vi "CVT Action Engine.vi"() -> ()   [LabVIEW 2021]
uses:
  CVT Command.ctl
  CVT Data Highway.ctl
  <vilib>/NI/Current Value Table/Current Value Table.lvlib
  <vilib>/NI/Current Value Table/Type Defs/Data Types.ctl
  <vilib>/NI/Current Value Table/Type Defs/Single Tag.ctl
  <vilib>/NI/Current Value Table/Type Defs/Tag Grouping set.ctl
  <vilib>/NI/Current Value Table/Type Defs/File Format.ctl
  <vilib>/NI/Current Value Table/DataTypes/Boolean_Write.vi
panel:
  in  "CVT Command":T1
  out "error out":errorcluster
  in  "error in (no error)":errorcluster
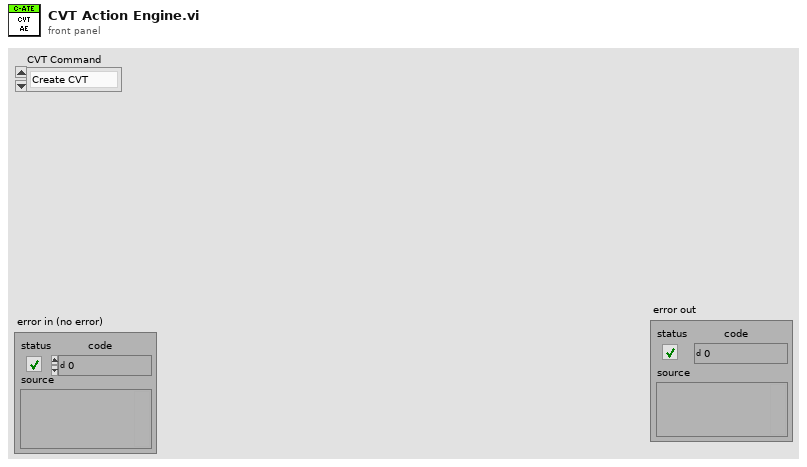
[diagram p1: front panel]
types:
  T1 = typedef "CVT Command.ctl" = enum16{"Create CVT", "Write Data ", "Read Data"}
  T2 = typedef "Current Value Table.lvlib/File Format.ctl" = cluster{"Tags":T3[], "Group Listings":T5[]}
  T3 = typedef "Current Value Table.lvlib/Single Tag.ctl" = cluster{"Data Type":T4, "Name":string, "Value":string, "Description":string}
  T4 = typedef "Current Value Table.lvlib/Data Types.ctl" = enum16{"Double", "Single", "I64", "I32", "I16", "I8", "U64", "U32", "U16", "U8", "String", "Boolean", "Array of U8", "Array of U16", "Array of U32", "Array of U64", "Array of I64", "Array of I32", "Array of I16", "Array of I8", "Array of Double", "Array of Single", "Array of Boolean", "Array of String"}
  T5 = typedef "Current Value Table.lvlib/Tag Grouping set.ctl" = cluster{"Group":string, "Tag Names":string[]}
  T6 = typedef "CVT Data Highway.ctl" = cluster{}
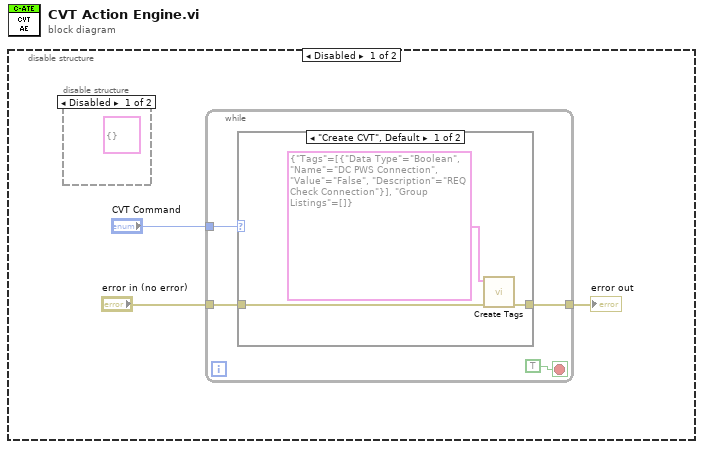
[diagram p0: block diagram]
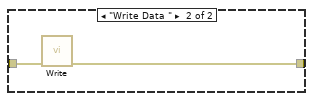
[diagram p3: hidden frame]
diagram:
  n1 = disable-structure shown="Disabled" {
    frame Disabled {
      n2 = disable-structure shown="Disabled" {
        frame Disabled {
          (unwired) T6 {}
        }
        frame Enabled {
        }
      }
      n3 = while {
        tunnel: "error in (no error)" -> [w6]
        tunnel: "CVT Command" -> [w5]
        tunnel: [w4] -> w1
        stop <- TRUE stop-if-true
        n4 = case shown="\"Create CVT\", Default" w5 {
          tunnel: w6 -> [w10 w12]
          tunnel: [w9 w11] -> w4
          frame "Create CVT", Default {
            n5 = call <vilib>:"Create Tags.vi"("error in (no error)"=w10, "CVT Tags to Create"=T2 {"Tags"=[{"Data Type"=enum."Boolean", "Name"="DC PWS Connection", "Value"="False", "Description"="REQ Check Connection"}], "Group Listings"=[]}) -> ("error out"=w9:errorcluster)  [unwired: 9 in]
          }
          frame "Write Data " {
            n6 = call-poly <vilib>:"Write.vi"("error in (no error)"=w12) -> ("error out"=w11:errorcluster)  [unwired: 10 in]
          }
        }
      }
      "error out" <- w1
    }
    frame Enabled {
    }
  }
